vi "checkSequenceIdRule.vi"(8 "error in (no error)":errorcluster, 10 "tcpPacket":string, 11 "tcpServerCmd in":refnum<class "TcpServerCmd.lvclass">) -> (0 "error out":errorcluster, 1 "ackIterations":i32, 2 "tcpPacket":string, 3 "tcpServerCmd out":refnum<class "TcpServerCmd.lvclass">)   [LabVIEW 2018, in "TcpServerCmd.lvclass"]
doc: "Get the sequence_id sent by TCP Client and compare it with lastSequenceId saved."
uses:
  TcpServerCmd.lvclass
  home/pcortes/github/ts_labview_tcp_json/src/TcpServerBase/TcpServerBase.lvclass
  TcpServerBase/TcpServerBase.lvclass/TcpServerBase.ctl
  TcpServerBase/TcpServerBase.lvclass
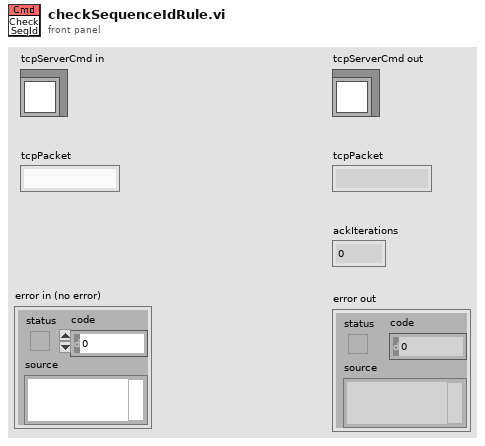
[diagram p1: front panel]
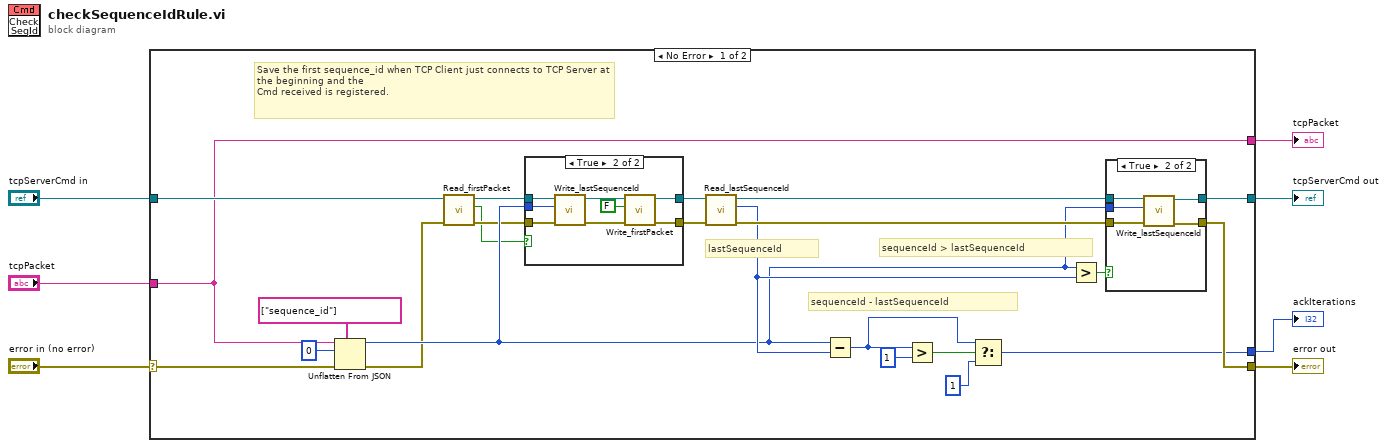
[diagram p0: block diagram]
diagram:
  n1 = case shown="No Error" "error in (no error)" {
    selector: "error in (no error)" -> [w28 w50]
    tunnel: [w25 w50] -> w6
    tunnel: "tcpServerCmd in" -> [w22 w49]
    tunnel: [w27 w49] -> w4
    tunnel: [w13 _] -> w3
    tunnel: "tcpPacket" -> [w8 w48]
    tunnel: [w8 w48] -> w1
    frame No Error {
      # "sequenceId > lastSequenceId"
      # "sequenceId - lastSequenceId"
      # "Save the first sequence_id when TCP Client just connects to TCP Server at the beginning and the\nCmd received is registered."
      # "lastSequenceId"
      n2 = Unflatten From JSON(path=string[] ["sequence_id"], JSON string=w8, type and defaults=0, error in (no error)=w28) -> (value=w15:i32, error out=w11:errorcluster)  [unwired: 3 in]
      n3 = call "Read_firstPacket.vi"("error in (no error)"=w11, "TcpServerBase in"=w22) -> ("error out"=w10:errorcluster, "firstPacket"=w9:bool, "TcpServerBase out"=w12:refnum<class "TcpServerCmd.lvclass">)  [unwired: 7 in]
      n4 = case shown="True" w9 {
        tunnel: w12 -> [w32 w40]
        tunnel: w15 -> [_ w37]
        tunnel: [w32 w34] -> w24
        tunnel: [w31 w36] -> w23
        tunnel: w10 -> [w31 w38]
        frame False {
        }
        frame True {
          n5 = call "Write_lastSequenceId.vi"("error in (no error)"=w38, "lastSequenceId"=w37, "TcpServerBase in"=w40) -> ("error out"=w39:errorcluster, "TcpServerBase out"=w35:refnum<class "TcpServerCmd.lvclass">)  [unwired: 7 in]
          n6 = call "Write_firstPacket.vi"("error in (no error)"=w39, "firstPacket"=FALSE, "TcpServerBase in"=w35) -> ("error out"=w36:errorcluster, "TcpServerBase out"=w34:refnum<class "TcpServerCmd.lvclass">)  [unwired: 7 in]
        }
      }
      n7 = call "Read_lastSequenceId.vi"("error in (no error)"=w23, "TcpServerBase in"=w24) -> ("error out"=w26:errorcluster, "lastSequenceId"=w16:i32, "TcpServerBase out"=w19:refnum<class "TcpServerCmd.lvclass">)  [unwired: 7 in]
      n8 = Subtract(x=w15, y=w16) -> (x-y=w17:i32)
      n9 = Greater?(x=w17, y=1) -> (0:w20:bool)
      n10 = Select(t=w17, s=w20, f=1) -> (s? t:f=w13:i32)
      n11 = Greater?(x=w15, y=w16) -> (0:w14:bool)
      n12 = case shown="True" w14 {
        tunnel: w19 -> [w42 w47]
        tunnel: [w42 w46] -> w27
        tunnel: w26 -> [w41 w45]
        tunnel: [w41 w44] -> w25
        tunnel: w15 -> [_ w43]
        frame False {
        }
        frame True {
          n13 = call "Write_lastSequenceId.vi"("error in (no error)"=w45, "lastSequenceId"=w43, "TcpServerBase in"=w47) -> ("error out"=w44:errorcluster, "TcpServerBase out"=w46:refnum<class "TcpServerCmd.lvclass">)  [unwired: 7 in]
        }
      }
    }
    frame Error {
    }
  }
  "error out" <- w6
  "tcpServerCmd out" <- w4
  "ackIterations" <- w3
  "tcpPacket" <- w1
